vi "LV to ITX 2D AutoPlot.vi"(4 "Notes":string, 6 "X,Y,Z Labels":string[](array[string])=["x", "y"], 8 "error in":errorcluster, 9 "Z Range":T1, 10 "2D, X, Y (Cluster)":T2, 11 "path":path) -> (0 "error out":errorcluster, 3 "file":path)   [LabVIEW 2019, in "LV-Data.ITX.lvclass"]
doc: "Write your 2D data to ITX file. This AutoPlot VI adds commands that will automatically create in Igor an intensity graph with X and Y axes scaled by the 1D arrays, allowing you to quickly view your data.\n\n-- path: base path to save data\n-- filename: base filename\n-- Notes: add any notes here to help you remember what experiment you did\n-- 2D Array: Intensity data\n-- X,Y Arrays: These are used to apply an appropriate scaling to the intensity graph\n-- X,Y wavenames: Default \"x_\" and \"y_\" are fine.\n-- X,Y,Z Labels: Labels for plotting in Igor."
uses:
  LV-Data.ITX.lvclass
  LV-Data/Typedefs/Operation--enum.ctl
  LV-Data/Typedefs/File Type--enum.ctl
  LV-Data/LV-Data.lvclass/LV-Data.ctl
  a931f469-99b5-40af-8282-0f943976f412.vi
  655ca478-e0df-4b9f-a929-c03e654f9e79.vi
  014960aa-8c2e-4c37-8344-5464a87ccff3.vi
  13c6573d-f149-4af1-bd30-f79d720bf89c.vi
  13c6573d-f149-4af1-bd30-f79d720bf89c.vi/d3d8ecf0-c0c0-44fe-a4c8-864ec08099fa.vi
  13c6573d-f149-4af1-bd30-f79d720bf89c.vi/9b10f1c8-2bce-4d71-a119-81829f20853c.vi
  <vilib>/AdvancedString/1D String Array to Delimited String.vi
  private/Variant to ITX Wave.vi
  private/Commands to ITX.vi
  private/Notes to ITX.vi
  LV-Data/LV-Data.lvclass
  ITX Commands/ITX Commands.lvclass
panel:
  # "Below are relevant for creating graphs in Igor"
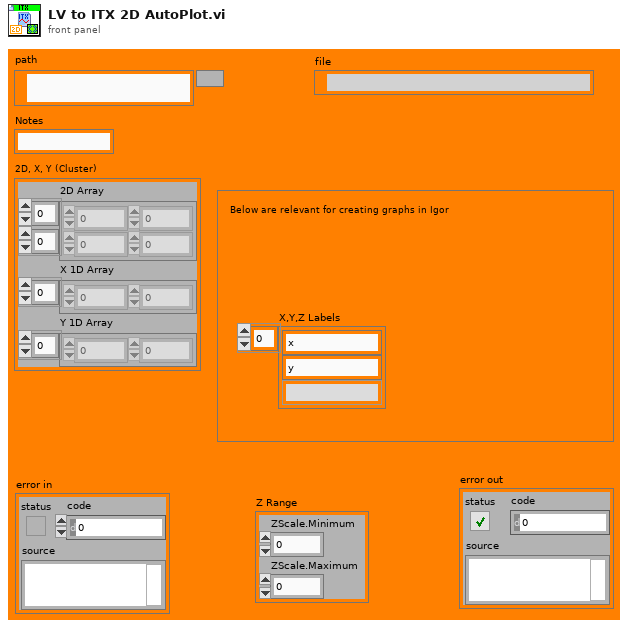
[diagram p1: front panel]
types:
  T1 = cluster{"ZScale.Minimum":dbl, "ZScale.Maximum":dbl}
  T2 = cluster{"2D Array":dbl[][], "X 1D Array":dbl[], "Y 1D Array":dbl[]}
  T3 = typedef "LV-Data.lvclass/File Type--enum.ctl" = enum16{"DAT", "ITX", "TDMS", "VI"}
  T4 = typedef "LV-Data.lvclass/Operation--enum.ctl" = enum16{"Read", "Write", "Write + Append"}
  T5 = typedef "LV-Data.lvclass/Map Variant--map.ctl" = map{string, variant}
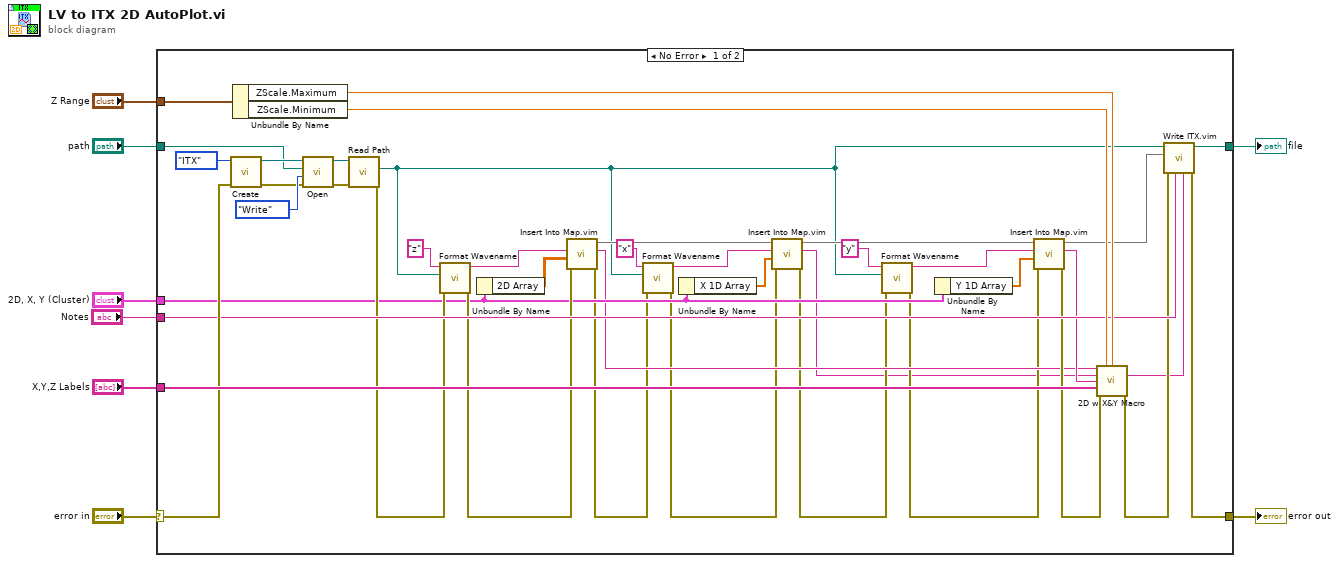
[diagram p0: block diagram]
diagram:
  n1 = case shown="No Error" "error in" {
    selector: "error in" -> [w37 w48]
    tunnel: "path" -> [w19 w47]
    tunnel: "Notes" -> [w34 _]
    tunnel: "X,Y,Z Labels" -> [w44 _]
    tunnel: [w29 w48] -> w5
    tunnel: [w35 w47] -> w4
    tunnel: "2D, X, Y (Cluster)" -> [w17 _]
    tunnel: "Z Range" -> [w43 _]
    frame No Error {
      n2 = call "Create.vi"("error in (no error)"=w37, "File Type"=File_Type--enum."ITX") -> ("error out"=w38:errorcluster, "Data out"=w39:refnum<class "LV-Data.lvclass">)  [unwired: 8 in]
      n3 = Unbundle By Name(w43) -> ("ZScale.Maximum"=w41:dbl, "ZScale.Minimum"=w42:dbl)
      n4 = call-dynamic "Open.vi"("error in (no error)"=w38, "Operation"=Operation--enum."Write", "Path"=w19, "Data in"=w39) -> ("error out"=w46:errorcluster, "Data out"=w45:refnum<class "LV-Data.lvclass">)  [unwired: 6 in]
      n5 = call "Read Path.vi"("error in (no error)"=w46, "Data Save"=w45) -> ("error out"=w27:errorcluster, "Path"=w9:path)  [unwired: 7 in, 1 out]
      n6 = call "Format Wavename.vi"("error in (no error)"=w27, "Path"=w9, "Name"="z") -> ("error out"=w26:errorcluster, "Formatted wavename"=w16:string)  [unwired: 7 in]
      n7 = Unbundle By Name(w17) -> ("2D Array"=w18:dbl[][])
      n8 = call "Insert Into Map.vim"("error in (no error)"=w26, "value"=w18, "key"=w16) -> ("error out"=w14:errorcluster, "map out"=w31:T5)  [unwired: 7 in]
      n9 = call "Format Wavename.vi"("error in (no error)"=w14, "Path"=w9, "Name"="x") -> ("error out"=w13:errorcluster, "Formatted wavename"=w10:string)  [unwired: 7 in]
      n10 = Unbundle By Name(w17) -> ("X 1D Array"=w15:dbl[])
      n11 = call "Insert Into Map.vim"("error in (no error)"=w13, "value"=w15, "key"=w10, "map in"=w31) -> ("error out"=w12:errorcluster, "map out"=w32:T5)  [unwired: 6 in]
      n12 = call "Format Wavename.vi"("error in (no error)"=w12, "Path"=w9, "Name"="y") -> ("error out"=w11:errorcluster, "Formatted wavename"=w23:string)  [unwired: 7 in]
      n13 = Unbundle By Name(w17) -> ("Y 1D Array"=w22:dbl[])
      n14 = call "Insert Into Map.vim"("error in (no error)"=w11, "value"=w22, "key"=w23, "map in"=w32) -> ("error out"=w33:errorcluster, "map out"=w21:T5)  [unwired: 6 in]
      n15 = call "2D w X&Y Macro.vi"("2D wave"=w16, "minimum"=w42, "maximum"=w41, "X wave"=w10, "Y wave"=w23, "X,Y,Z Labels"=w44, "error in (no error)"=w33) -> ("result string"=w20:string, "error out"=w30:errorcluster)  [unwired: 6 in, 1 out]
      n16 = call "Write ITX.vim"("commands"=w20, "notes"=w34, "error in"=w30, "values"=w21, "filename"=w9) -> ("error out"=w29:errorcluster, "filename out"=w35:path)  [unwired: 4 in, 1 out]
    }
    frame Error {
    }
  }
  "file" <- w4
  "error out" <- w5
